vi "DSF.Engine.Memory.ObjectPool.Return Index.vi"(8 "error in (no error)":errorcluster, 9 "timeout ms (0)":i32 format="%d ms", 10 "index":i32, 11 "ObjectPool in":refnum<class "DSF.Engine.Memory.ObjectPool.lvclass">) -> (0 "error out":errorcluster, 1 "timed out?":bool, 3 "ObjectPool out":refnum<class "DSF.Engine.Memory.ObjectPool.lvclass">)   [LabVIEW 2016, in "DSF.Engine.lvlib" / "DSF.Engine.Memory.ObjectPool.lvclass"]
uses:
  DSF.Engine.Memory.ObjectPool.lvclass
  DSF.Engine.Memory.ObjectPool.lvclass/DSF.Engine.Memory.ObjectPool.ctl
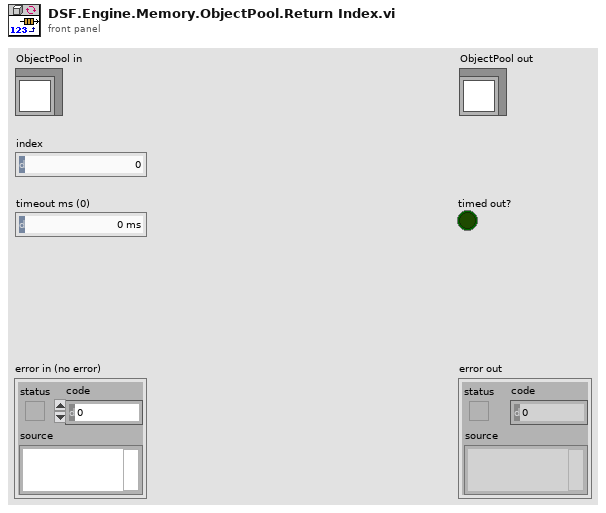
[diagram p1: front panel]
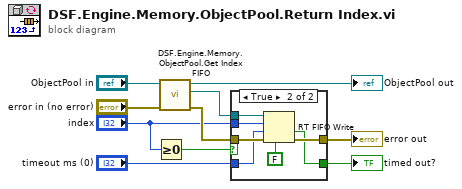
[diagram p0: block diagram]
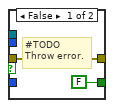
[diagram p2: hidden frame]
diagram:
  n1 = Greater Or Equal To 0?(x="index") -> (x >= 0?=w2:bool)
  n2 = call "DSF.Engine.Memory.ObjectPool.Get Index FIFO.vi"("error in (no error)"="error in (no error)", "ObjectPool in"="ObjectPool in") -> ("error out"=w7:errorcluster, "Index FIFO"=w8:refnum<k33>, "ObjectPool out"=→"ObjectPool out":refnum<class "DSF.Engine.Memory.ObjectPool.lvclass">)  [unwired: 7 in]
  n3 = case shown="True" w2 {
    tunnel: w8 -> [_ w19]
    tunnel: w7 -> [w11 w18]
    tunnel: [w11 w16] -> w6
    tunnel: "timeout ms (0)" -> [_ w15]
    tunnel: [FALSE ("timed out?") w14] -> w4
    tunnel: "index" -> [_ w13]
    frame False {
      # "#TODO\nThrow error."
    }
    frame True {
      n4 = RT FIFO Write(0:w19, 1:w13, 2:w15, 3:w18, 5:FALSE ("overwrite on timeout (T)")) -> (10:w14:bool, 11:w16:errorcluster)  [unwired: 2 out]
    }
  }
  "error out" <- w6
  "timed out?" <- w4
